vi "SafeModeFilter.vi"(11 "action in":string) -> (3 "action out":string)   [LabVIEW 2017, in "Qbus.lvclass"]
uses:
  <vilib>/addons/Qbus/Qbus.lvclass
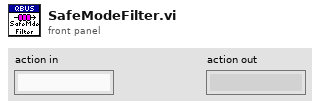
[diagram p1: front panel]
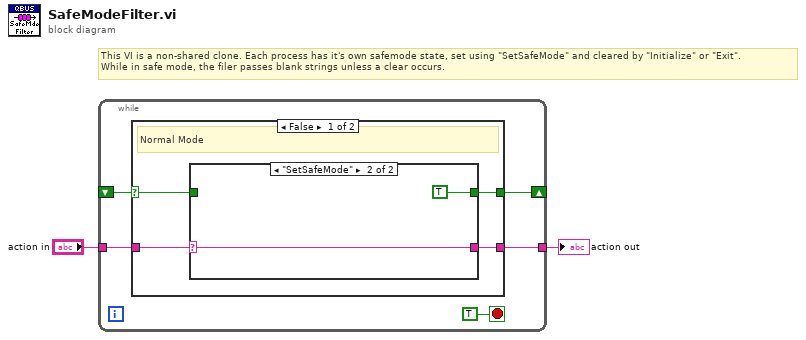
[diagram p0: block diagram]
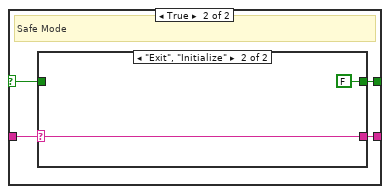
[diagram p3: hidden frame]
diagram:
  # "This VI is a non-shared clone. Each process has it's own safemode state, set using \"SetSafeMode\" and cleared by \"Initialize\" or \"Exit\". \nWhile in safe mode, the filer passes blank strings unless a clear occurs."
  n1 = while {
    tunnel: "action in" -> [w6]
    tunnel: [w5] -> w1
    shift-right: [w3] -> _
    shift-left: _ -> [w4]
    stop <- TRUE stop-if-true
    n2 = case shown="False" w4 {
      selector: w4 -> [w8 w19]
      tunnel: [w10 w17] -> w5
      tunnel: [w9 w16] -> w3
      tunnel: w6 -> [w11 w18]
      frame False {
        # "Normal Mode"
        n3 = case shown="\"SetSafeMode\"" w11 {
          selector: w11 -> [w12 w15]
          tunnel: [w12 w15] -> w10
          tunnel: [w13 TRUE] -> w9
          tunnel: w8 -> [w13 _]
          frame Default {
          }
          frame "SetSafeMode" {
          }
        }
      }
      frame True {
        # "Safe Mode"
        n4 = case shown="\"Exit\", \"Initialize\"" w18 {
          selector: w18 -> [_ w22]
          tunnel: [_ w22] -> w17
          tunnel: [w20 FALSE] -> w16
          tunnel: w19 -> [w20 _]
          frame Default {
          }
          frame "Exit", "Initialize" {
          }
        }
      }
    }
  }
  "action out" <- w1
